vi "Error - Tests.vi"(8 "error in (no error)":errorcluster) -> (0 "error out":errorcluster)   [LabVIEW 2017]
uses:
  System.Windows.Forms
  <vilib>/addons/_JKI Toolkits/Caraya/classes/Assert/Assert Error.vi
  <vilib>/addons/_JKI Toolkits/Caraya/classes/Assert/Assert Equal Value_Variant.vi
  <vilib>/addons/_JKI Toolkits/Caraya/classes/Test/Test.lvclass
  <vilib>/addons/_JKI Toolkits/Caraya/classes/Assert/Assert.lvclass
  src/Error Dialog w Copy to Clipboard.lvlib
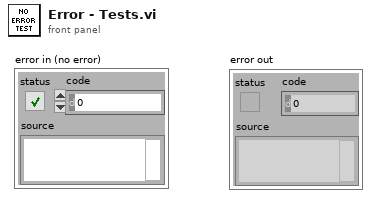
[diagram p1: front panel]
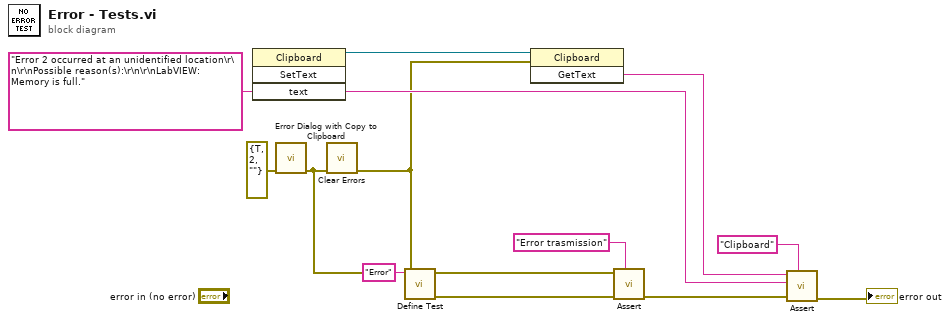
[diagram p0: block diagram]
diagram:
  w5 = "Error 2 occurred at an unidentified location\r\n\r\nPossible reason(s):\r\n\r\nLabVIEW:  Memory is full." ("text")
  n1 = invoke class="Clipboard" method="SetText"("text"=w5) -> (reference out=w8:refnum<k24>)  [unwired: 3 in, 3 out]
  n2 = call "Error Dialog with Copy to Clipboard.vi"("error in (no error)"=errorcluster {"status"=TRUE, "code"=2, "source"=""}) -> ("error out"=w1:errorcluster)  [unwired: 10 in]
  n3 = call <vilib>:"Clear Errors.vi"("error in (no error)"=w1) -> ("error out"=w2:errorcluster)  [unwired: 5 in, 1 out]
  n4 = call <vilib>:"Define Test.vi"("error in (no error)"=w2, "Label (VI Title)"="Error") -> ("error out"=w10:errorcluster)  [unwired: 9 in]
  n5 = invoke class="Clipboard" method="GetText"(reference=w8, error in=w2) -> ("GetText"=w6:string)  [unwired: 1 in, 2 out]
  n6 = call-poly <vilib>:"Assert.vi"("Label"="Error trasmission", "error in (no error)"=w10, "Error?"=w1) -> ("error out"=w7:errorcluster)  [unwired: 8 in]
  n7 = call-poly <vilib>:"Assert.vi"("Label"="Clipboard", "error in (no error)"=w7, "Y"=w5, "X"=w6) -> ("error out"=→"error out":errorcluster)  [unwired: 7 in]
